vi "Setup UI.vi"(8 "error in (no error)":errorcluster, 10 "Set UI to input? (F)":bool, 11 "Wavelength iHR320 in":refnum<class "Wavelength iHR320.lvclass">) -> (0 "error out":errorcluster, 3 "Wavelength iHR320 out":refnum<class "Wavelength iHR320.lvclass">)   [LabVIEW 2009, in "Wavelength iHR320.lvclass"]
doc: "Scanner::Setup is a constructor that has no parameters and faces the user. The Factory calls this VI to let the user configure this Scanner. It is dynamically dispatched in order to let the user choose the type as well as the options of the scanner."
uses:
  Wavelength iHR320.lvclass
  Wavelength iHR320.lvclass/Wavelength iHR320.ctl
panel:
  out "Step Size":dbl
  in  "Front Exit":dbl[unit]
  in  "Front Entrance":dbl[unit]
  # "iHR 320 Wavelength"
  # "Needs to be checked!"
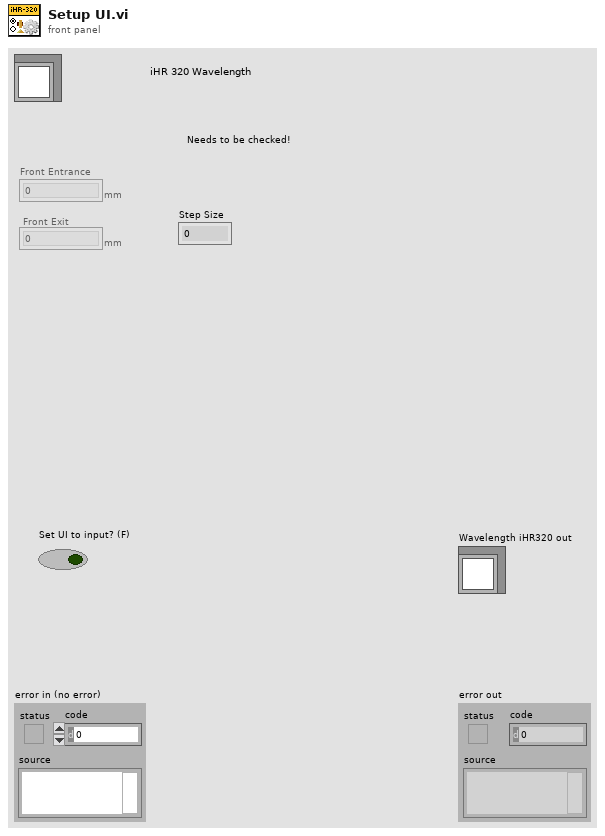
[diagram p1: front panel]
types:
  T1 = typedef "Scanner.lvclass/Range.ctl" = cluster{"xi":dbl, "xf":dbl, "dx":dbl, "Return to...?":bool, "Return to":dbl}
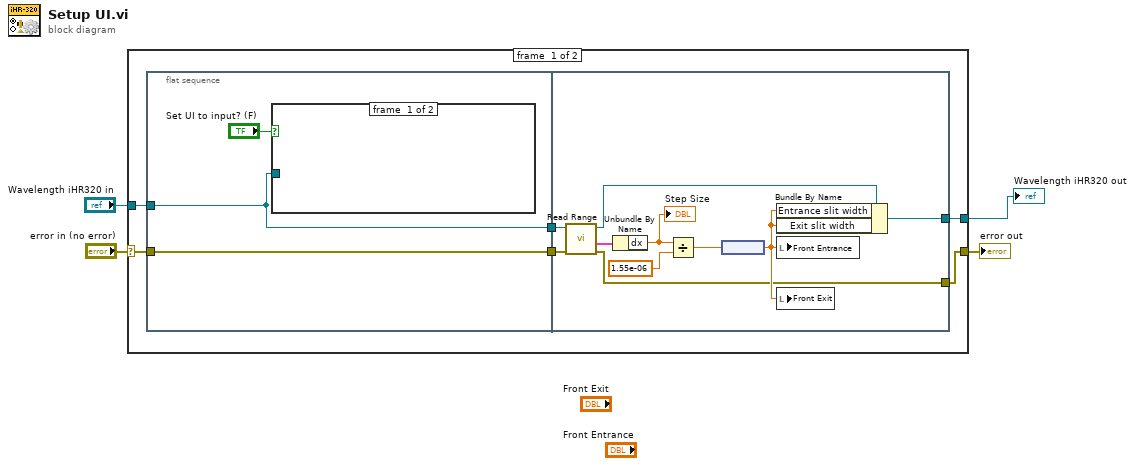
[diagram p0: block diagram]
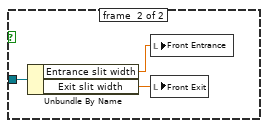
[diagram p2: hidden frame]
diagram:
  n1 = case shown="No Error" "error in (no error)" {
    selector: "error in (no error)" -> [w7 w28]
    tunnel: [w5 w28] -> w3
    tunnel: "Wavelength iHR320 in" -> [w10 w27]
    tunnel: [w6 w27] -> w1
    frame #0 {
      n2 = flat-sequence {
        tunnel: w10 -> [w12]
        tunnel: [w12] -> w9
        tunnel: [w11] -> w8
        tunnel: w7 -> [w11]
        tunnel: w9 -> [w26]
        tunnel: w8 -> [w25]
        tunnel: [w18] -> w6
        tunnel: [w17] -> w5
        frame #0 {
          n3 = case shown="True" "Set UI to input? (F)" {
            tunnel: w12 -> [_ w16]
            frame #0 {
            }
            frame #1 {
              n4 = Unbundle By Name(w16) -> ("Entrance slit width"=w15:dbl[unit], "Exit slit width"=w14:dbl[unit])
              n5 = local write "Front Entrance"(w15) -> ()
              n6 = local write "Front Exit"(w14) -> ()
            }
          }
        }
        frame #1 {
          n7 = call-dynamic "Read Range.vi"("error in (no error)"=w25, "Scanner.lvclass in"=w26) -> ("error out"=w17:errorcluster, "Range"=w24:T1, "Scanner.lvclass out"=w20:refnum<class "Wavelength iHR320.lvclass">)  [unwired: 4 in, 3 out]
          n8 = Unbundle By Name(w24) -> ("dx"=w23:dbl)
          "Step Size" <- w23
          n9 = Divide(x=w23, y=1.55e-06) -> (x/y=w21:dbl)
          n10 = node(w21) -> (w19:dbl[unit])
          n11 = Bundle By Name(cluster=w20, "Entrance slit width"=w19, "Exit slit width"=w19) -> (w18:refnum<class "Wavelength iHR320.lvclass">)
          n12 = local write "Front Entrance"(w19) -> ()
          n13 = local write "Front Exit"(w19) -> ()
        }
      }
    }
    frame #1 {
    }
  }
  "error out" <- w3
  "Wavelength iHR320 out" <- w1
